vi "Get Default Ephemeral Strategies.vi"(10 "Ephemeral Strategies in":map{string, refnum<class "BananaPeel.lvclass">}(c390)) -> (2 "Ephemeral Strategies":map{string, refnum<class "BananaPeel.lvclass">}(c390))   [LabVIEW 2021, in "Bananas.lvlib" / "Platano.lvclass"]
uses:
  BananaPeel/BananaPeel.lvclass
  Assertion Strategies -- cluster.ctl
  AssertTrue/AssertTrue.lvclass
  AssertFalse/AssertFalse.lvclass
  AssertEqualValue/AssertEqualValue.lvclass
  AssertEqualType/AssertEqualType.lvclass
  AssertCompareValue/AssertCompareValue.lvclass
  AssetError/AssertError.lvclass
  AssertAlmostEqual/AssertAlmostEqualValue.lvclass
  Test Strategies -- cluster.ctl
  DefineTest/DefineTest.lvclass
  DefineSuite/DefineSuite.lvclass
  <vilib>/LabVIEW Open Source Project/Data Manipulation/TypeDescriptor/TypeDescriptor_GetName.vi
  <vilib>/LabVIEW Open Source Project/Data Manipulation/TypeDescriptor/TypeDescriptor_GetType.vi
  <vilib>/LabVIEW Open Source Project/Data Manipulation/TypeDescriptor/TypeDescriptor_GetPString.vi
  Platano/Platano.lvclass
  Bananas.lvlib
  <vilib>/LabVIEW Open Source Project/Data Manipulation/Variant/OpenVariant.lvlib
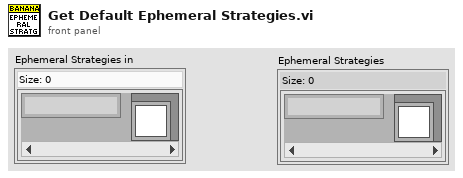
[diagram p1: front panel]
types:
  T1 = typedef "Bananas.lvlib/Test Strategies -- cluster.ctl" = cluster{"DefineTest":refnum<class "DefineTest.lvclass">, "DefineSuite":refnum<class "DefineSuite.lvclass">}
  T2 = typedef "Bananas.lvlib/Assertion Strategies -- cluster.ctl" = cluster{"AssertTrue":refnum<class "AssertTrue.lvclass">, "AssertFalse":refnum<class "AssertFalse.lvclass">, "AssertEqualValue":refnum<class "AssertEqualValue.lvclass">, "AssertEqualType":refnum<class "AssertEqualType.lvclass">, "AssertCompareValue":refnum<class "AssertCompareValue.lvclass">, "AssertError":refnum<class "AssertError.lvclass">, "AssertAlmostEqual":refnum<class "AssertAlmostEqualValue.lvclass">}
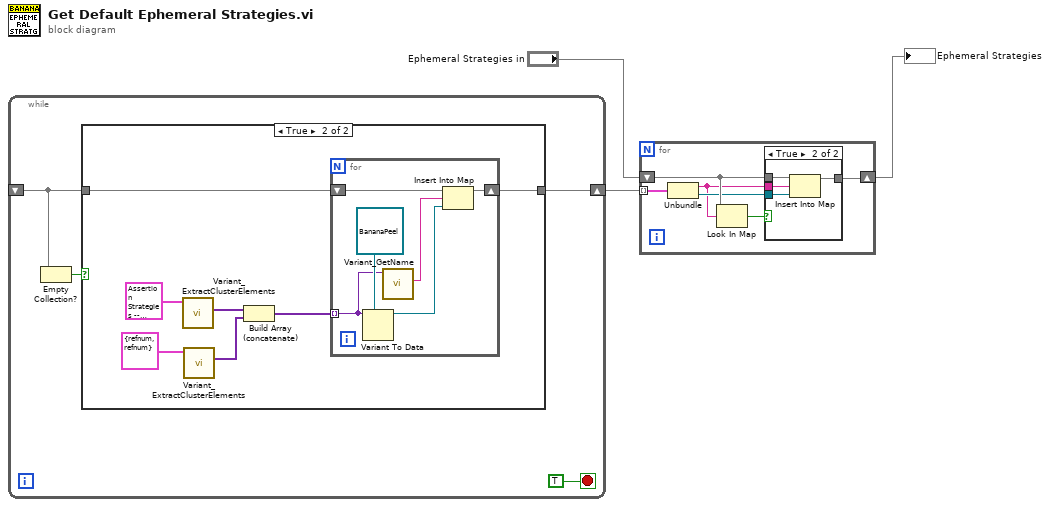
[diagram p0: block diagram]
diagram:
  n1 = while {
    shift-right: [w5] -> w1
    shift-left: _ -> [w6]
    stop <- TRUE stop-if-true
    n2 = Empty Collection?(1:w6) -> (0:w7:bool)
    n3 = case shown="True" w7 {
      tunnel: w6 -> [w8 w14]
      tunnel: [w8 w13] -> w5
      frame False {
      }
      frame True {
        n4 = call <vilib>:"Variant_ExtractClusterElements.vi"("Cluster"=T2 {"AssertTrue"=refnum, "AssertFalse"=refnum, "AssertEqualValue"=refnum, "AssertEqualType"=refnum, "AssertCompareValue"=refnum, "AssertError"=refnum, "AssertAlmostEqual"=refnum} ("Strategies")) -> ("Elements"=w10:variant[])  [unwired: 8 in, 2 out]
        n5 = call <vilib>:"Variant_ExtractClusterElements.vi"("Cluster"=T1 {"DefineTest"=refnum, "DefineSuite"=refnum} ("Strategies 2")) -> ("Elements"=w11:variant[])  [unwired: 8 in, 2 out]
        n6 = Build Array (concatenate)(w10, w11) -> (w9:variant[])
        n7 = for {
          tunnel: w9 -> [w20] mode=indexing
          shift-right: [w19] -> w13
          shift-left: w14 -> [w18]
          n8 = Variant To Data(type=refnum<class "BananaPeel.lvclass"> refnum ("BananaPeel"), Variant=w20) -> (data=w16:refnum<class "BananaPeel.lvclass">)  [unwired: 1 in, 1 out]
          n9 = call <vilib>:"Variant_GetName.vi"("Variant"=w20) -> ("Name"=w17:string)  [unwired: 8 in, 2 out]
          n10 = Insert Into Map(map in=w18, key=w17, value=w16) -> (map out=w19:map{string, refnum<class "BananaPeel.lvclass">})  [unwired: 2 out]
        }
      }
    }
  }
  n11 = for {
    shift-right: [w26] -> w3
    shift-left: "Ephemeral Strategies in" -> [w27]
    tunnel: w1 -> [w24] mode=indexing
    n12 = Unbundle(w24) -> ("Name"=w22:string, "BananaPeel"=w23:refnum<class "BananaPeel.lvclass">)
    n13 = Look In Map(map=w27, key=w22) -> (key not found?=w25:bool)  [unwired: 1 in, 1 out]
    n14 = case shown="True" w25 {
      tunnel: w27 -> [w28 w32]
      tunnel: [w28 w31] -> w26
      tunnel: w22 -> [_ w30]
      tunnel: w23 -> [_ w29]
      frame False {
      }
      frame True {
        n15 = Insert Into Map(map in=w32, key=w30, value=w29) -> (map out=w31:map{string, refnum<class "BananaPeel.lvclass">})  [unwired: 2 out]
      }
    }
  }
  "Ephemeral Strategies" <- w3
